vi "File.Config, List Sections and Items in an INI File.vi"(8 "error in (no error)":errorcluster, 11 "Path":path) -> (0 "error out":errorcluster, 3 "Items":string[][](array[string]))   [LabVIEW 2018]
uses:
  <vilib>/Utility/config.llb/NI_LVConfig.lvlib
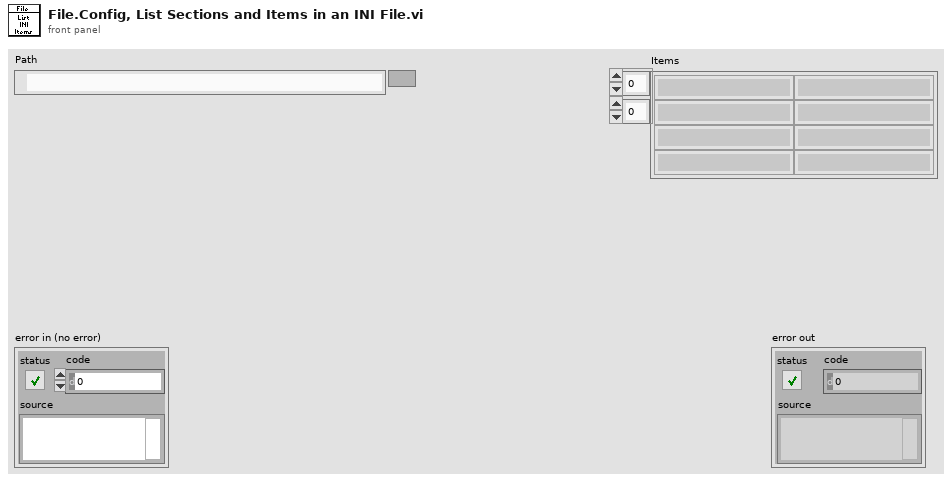
[diagram p1: front panel]
types:
  T1 = typedef "NI_LVConfig.lvlib/Config Data RefNum.ctl" = refnum<k1>
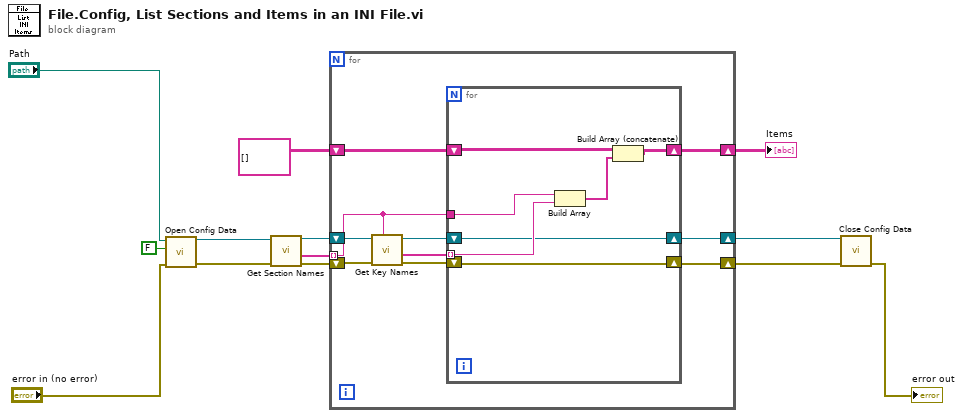
[diagram p0: block diagram]
diagram:
  n1 = call <vilib>:"Open Config Data.vi"("error in (no error)"="error in (no error)", "create file if necessary (T)"=FALSE, "configuration file path"="Path") -> ("error out"=w10:errorcluster, "refnum"=w11:T1)  [unwired: 6 in, 1 out]
  n2 = call <vilib>:"Get Section Names.vi"("error in (no error)"=w10, "refnum"=w11) -> ("error out"=w6:errorcluster, "section names"=w9:string[], "refnum out"=w7:T1)  [unwired: 7 in]
  n3 = for {
    tunnel: w9 -> [w17] mode=indexing
    shift-right: [w14] -> w2
    shift-left: string[][] [] -> [w19]
    shift-right: [w16] -> w5
    shift-left: w7 -> [w23]
    shift-right: [w15] -> w3
    shift-left: w6 -> [w22]
    n4 = call <vilib>:"Get Key Names.vi"("section"=w17, "error in (no error)"=w22, "refnum"=w23) -> ("error out"=w21:errorcluster, "key names"=w18:string[], "refnum out"=w20:T1)  [unwired: 5 in, 1 out]
    n5 = for {
      shift-right: [w28] -> w16
      shift-left: w20 -> [w28]
      shift-right: [w24] -> w14
      shift-left: w19 -> [w26]
      tunnel: w18 -> [w29] mode=indexing
      tunnel: w17 -> [w30]
      shift-right: [w27] -> w15
      shift-left: w21 -> [w27]
      n6 = Build Array(w30, w29) -> (w25:string[])
      n7 = Build Array (concatenate)(w26, w25) -> (w24:string[][])
    }
  }
  "Items" <- w2
  n8 = call <vilib>:"Close Config Data.vi"("error in (no error)"=w3, "refnum"=w5) -> ("error out"=→"error out":errorcluster)  [unwired: 8 in, 1 out]
